vi "Set Control by Name.vi"(6 "signaling (T)":bool=TRUE, 8 "error in (no error)":errorcluster, 9 "value":variant, 10 "control name":string, 11 "vi name":string) -> (0 "error out":errorcluster)   [LabVIEW 2018, in "STEPkgDriver_LINC.lvlib"]
uses:
  STEPkgDriver_LINC.lvlib
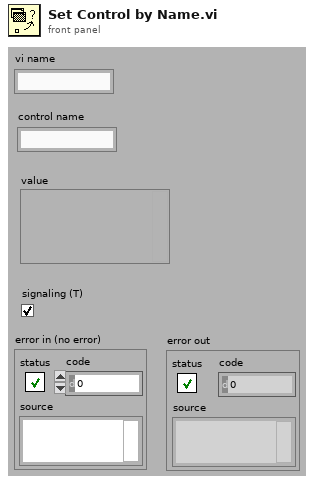
[diagram p1: front panel]
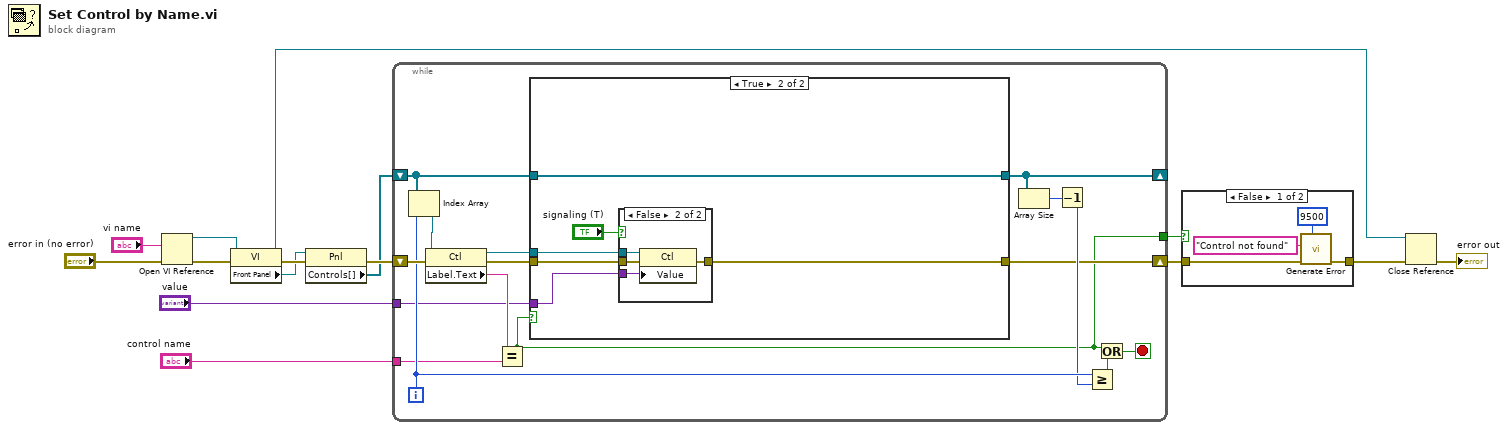
[diagram p0: block diagram]
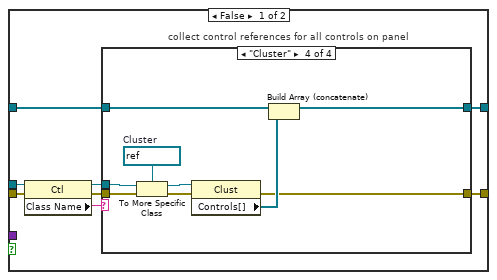
[diagram p3: hidden frame]
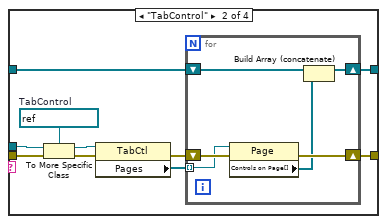
[diagram p5: hidden frame]
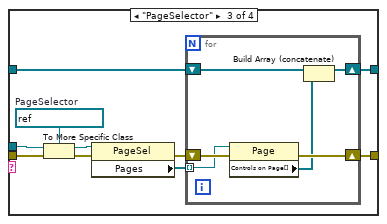
[diagram p6: hidden frame]
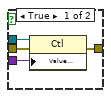
[diagram p7: hidden frame]
diagram:
  n1 = Open VI Reference(vi path="vi name", error in (no error)="error in (no error)") -> (vi reference=w15:refnum<vi>, error out=w14:errorcluster)  [unwired: 4 in]
  n2 = property class="VI"(reference=w15, error in=w14) -> (reference out=w13:refnum<vi>, error out=w6:errorcluster, "Front Panel"=w5:refnum<vi>)
  n3 = property class="Pnl"(reference=w5, error in=w6) -> (error out=w4:errorcluster, "Controls[]"=w3:refnum<vi>[])  [unwired: 1 out]
  n4 = while {
    shift-right: [w19] -> w2
    shift-left: w4 -> [w31]
    shift-right: [w20] -> _
    shift-left: w3 -> [w21]
    tunnel: "control name" -> [w18]
    tunnel: "value" -> [w17]
    tunnel: [w16] -> w1
    i -> [w28]
    stop <- w22 stop-if-true
    n5 = Index Array(array=w21, index=w28) -> (element=w30:refnum<vi>)
    n6 = property class="Ctl"(reference=w30, error in=w31) -> (reference out=w24:refnum<vi>, error out=w25:errorcluster, "Label.Text"=w26:string)
    n7 = Equal?(x=w26, y=w18) -> (x = y?=w16:bool)
    n8 = case shown="True" w16 {
      tunnel: w25 -> [w35 w88]
      tunnel: w24 -> [w36 w87]
      tunnel: [w39 w86] -> w19
      tunnel: w21 -> [w38 w85]
      tunnel: [w37 w85] -> w20
      tunnel: w17 -> [_ w84]
      frame False {
        # "collect control references for all controls on panel"
        n9 = property class="Ctl"(reference=w36, error in=w35) -> (reference out=w32:refnum<vi>, error out=w33:errorcluster, "Class Name"=w34:string)
        n10 = case shown="\"Cluster\"" w34 {
          tunnel: w33 -> [w41 w50 w66 w81]
          tunnel: w32 -> [_ w51 w67 w82]
          tunnel: w38 -> [w40 w44 w60 w77]
          tunnel: [w41 w43 w59 w74] -> w39
          tunnel: [w40 w42 w58 w76] -> w37
          frame Default {
          }
          frame "TabControl" {
            w47 = refnum<vi> refnum  # TabControl
            n11 = To More Specific Class(target class=w47, reference=w51, error in=w50) -> (specific class reference=w48:refnum<vi>, error out=w49:errorcluster)
            n12 = property class="TabCtl"(reference=w48, error in=w49) -> (error out=w46:errorcluster, "Pages"=w45:refnum<vi>[])  [unwired: 1 out]
            n13 = for {
              shift-right: [w55] -> w43
              shift-left: w46 -> [w57]
              tunnel: w45 -> [w56] mode=indexing
              shift-right: [w52] -> w42
              shift-left: w44 -> [w54]
              n14 = property class="Page"(reference=w56, error in=w57) -> (error out=w55:errorcluster, "Controls on Page[]"=w53:refnum<vi>[])  [unwired: 1 out]
              n15 = Build Array (concatenate)(w54, w53) -> (w52:refnum<vi>[])
            }
          }
          frame "PageSelector" {
            w63 = refnum<vi> refnum  # PageSelector
            n16 = To More Specific Class(target class=w63, reference=w67, error in=w66) -> (specific class reference=w64:refnum<vi>, error out=w65:errorcluster)
            n17 = property class="PageSel"(reference=w64, error in=w65) -> (error out=w62:errorcluster, "Pages"=w61:refnum<vi>[])  [unwired: 1 out]
            n18 = for {
              shift-right: [w71] -> w59
              shift-left: w62 -> [w73]
              tunnel: w61 -> [w72] mode=indexing
              shift-right: [w68] -> w58
              shift-left: w60 -> [w70]
              n19 = property class="Page"(reference=w72, error in=w73) -> (error out=w71:errorcluster, "Controls on Page[]"=w69:refnum<vi>[])  [unwired: 1 out]
              n20 = Build Array (concatenate)(w70, w69) -> (w68:refnum<vi>[])
            }
          }
          frame "Cluster" {
            w78 = refnum<vi> refnum  # Cluster
            n21 = To More Specific Class(target class=w78, reference=w82, error in=w81) -> (specific class reference=w79:refnum<vi>, error out=w80:errorcluster)
            n22 = property class="Clust"(reference=w79, error in=w80) -> (error out=w74:errorcluster, "Controls[]"=w75:refnum<vi>[])  [unwired: 1 out]
            n23 = Build Array (concatenate)(w77, w75) -> (w76:refnum<vi>[])
          }
        }
      }
      frame True {
        n24 = case shown="False" "signaling (T)" {
          tunnel: w88 -> [w92 w96]
          tunnel: w87 -> [w91 w95]
          tunnel: [w90 w94] -> w86
          tunnel: w84 -> [w89 w93]
          frame True {
            n25 = property class="Ctl"(reference=w91, error in=w92, "Value (Signaling)"=w89) -> (error out=w90:errorcluster)  [unwired: 1 out]
          }
          frame False {
            n26 = property class="Ctl"(reference=w95, error in=w96, "Value"=w93) -> (error out=w94:errorcluster)  [unwired: 1 out]
          }
        }
      }
    }
    n27 = Array Size(array=w20) -> (size(s)=w29:i32)
    n28 = Decrement(x=w29) -> (x-1=w27:i32)
    n29 = Greater Or Equal?(x=w28, y=w27) -> (x >= y?=w23:bool)
    n30 = Or(x=w16, y=w23) -> (x .or. y?=w22:bool)
  }
  n31 = case shown="False" w1 {
    tunnel: w2 -> [w100 w101]
    tunnel: [w99 w101] -> w9
    frame False {
      n32 = call "Generate Error.vi"("error code (-1301)"=9500, "error in"=w100, "description"="Control not found") -> ("error out"=w99:errorcluster)  [unwired: 8 in]
    }
    frame True {
    }
  }
  n33 = Close Reference(reference=w13, error in (no error)=w9) -> (error out=→"error out":errorcluster)
